vi "KE622x -- Set List Sweep Steps.vi"(0 "Resource In":refnum<visa-resource-name>, 1 "Check For SCPI Errors? (T)":bool=TRUE, 7 "List Sweep Steps In":T1 {"Current Level (A)" min=-0.105 max=0.105 format="%.4p"; "Source Delay (s)" min=0.001 max=1000.0 step=0.001 format="%.3f"; "Voltage Limit (V)" min=0.1 max=105.0 step=0.01 format="%.2p"}, 11 "error in (no error)":errorcluster, 12 "Read Back Set Values? (T)":bool=TRUE) -> (4 "Resource Out (dupl)":refnum<visa-resource-name>, 8 "List Sweep Steps Out":T1 {"Current Level (A)" min=-0.105 max=0.105 format="%.4p"; "Source Delay (s)" min=0.001 max=1000.0 step=0.001 format="%.3f"; "Voltage Limit (V)" min=0.1 max=105.0 step=0.01 format="%.2p"}, 15 "error out":errorcluster)   [LabVIEW 2019, in "Keithley 622x.lvlib"]
doc: "Sets up the individual points in a list current sweep."
uses:
  Keithley 622x.lvlib
  Typedefs/KE622x -- List Sweep Steps.ctl
  Typedefs/KE622x -- List Sweep Step.ctl
  Typedefs/KE622x -- Current Level.ctl
  Typedefs/KE622x -- Source Delay.ctl
  Typedefs/KE622x -- Voltage Limit.ctl
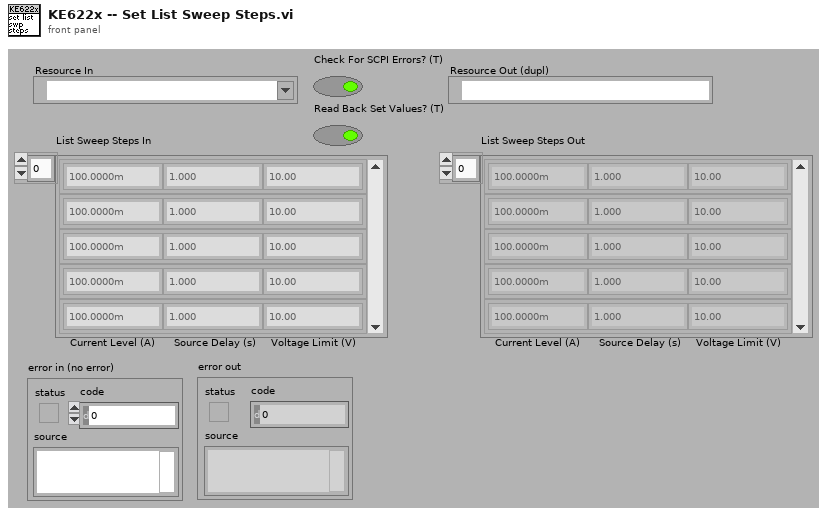
[diagram p1: front panel]
types:
  T1 = typedef "Keithley 622x.lvlib/KE622x -- List Sweep Steps.ctl" = T2[]
  T2 = typedef "Keithley 622x.lvlib/KE622x -- List Sweep Step.ctl" = cluster{"Current Level (A)":T3, "Source Delay (s)":T4, "Voltage Limit (V)":T5}
  T3 = typedef "Keithley 622x.lvlib/KE622x -- Current Level.ctl" = dbl
  T4 = typedef "Keithley 622x.lvlib/KE622x -- Source Delay.ctl" = dbl
  T5 = typedef "Keithley 622x.lvlib/KE622x -- Voltage Limit.ctl" = dbl
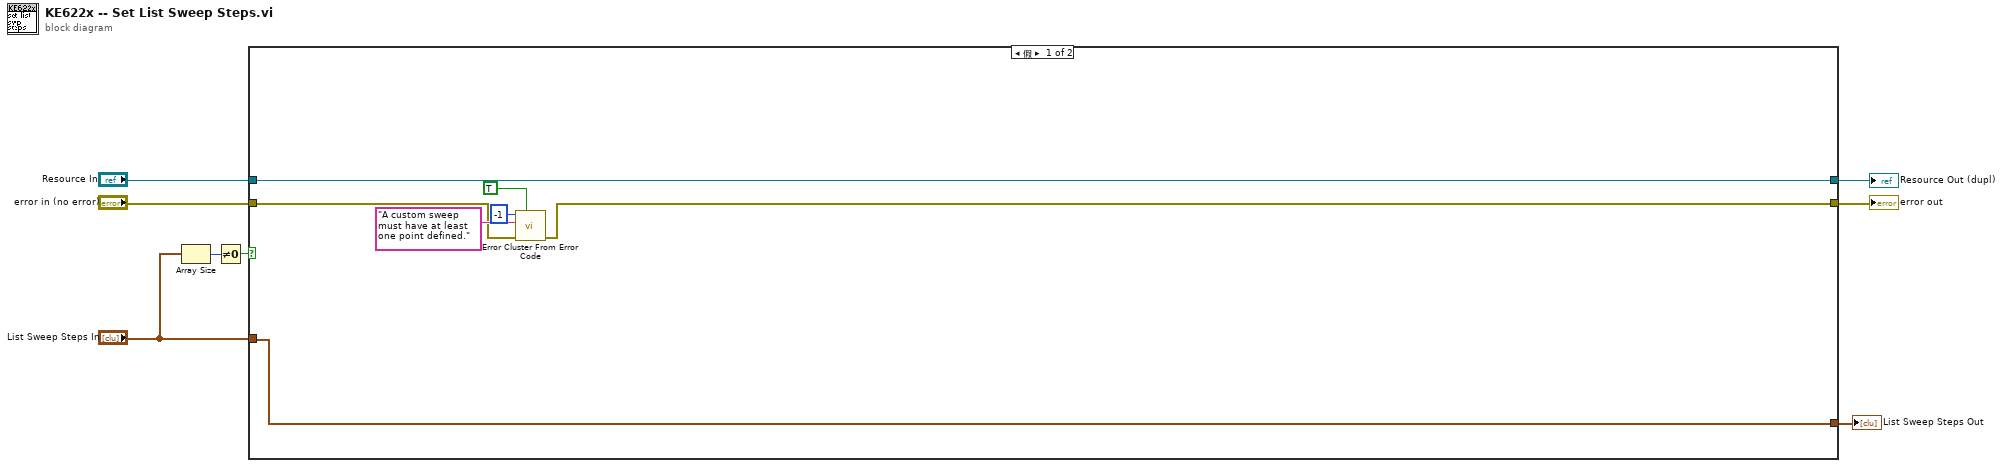
[diagram p0: block diagram]
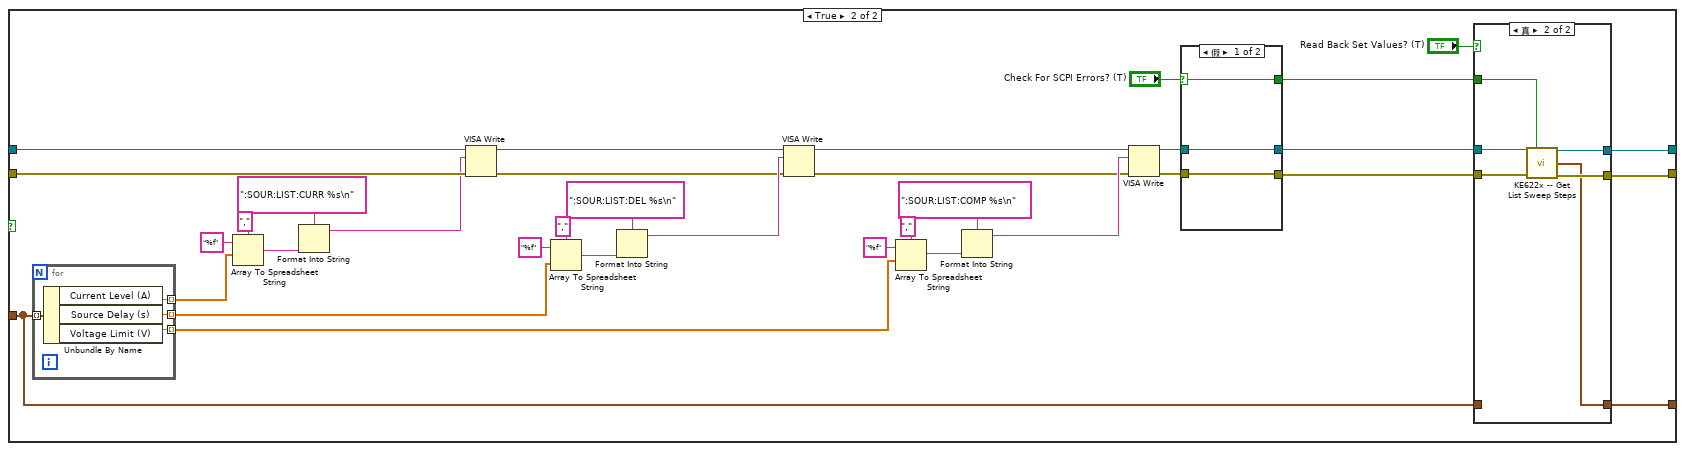
[diagram p2: hidden frame]
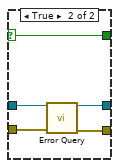
[diagram p4: hidden frame]
diagram:
  n1 = Array Size(array="List Sweep Steps In") -> (size(s)=w6:i32)
  n2 = Not Equal To 0?(x=w6) -> (x != 0?=w5:bool)
  n3 = case shown="假" w5 {
    tunnel: "List Sweep Steps In" -> [w14 w22]
    tunnel: "Resource In" -> [w15 w48]
    tunnel: "error in (no error)" -> [w11 w47]
    tunnel: [w15 w18] -> w3
    tunnel: [w9 w17] -> w2
    tunnel: [w14 w16] -> w1
    frame False {
      n4 = call <vilib>:"Error Cluster From Error Code.vi"("show call chain? (False)"=TRUE, "error in (no error)"=w11, "error message (\"\")"="A custom sweep must have at least one point defined.", "error code (0)"=-1) -> ("error out"=w9:errorcluster)  [unwired: 5 in]
    }
    frame True {
      n5 = for {
        tunnel: w22 -> [w71] mode=indexing
        tunnel: [w70] -> w49 mode=indexing
        tunnel: [w69] -> w38 mode=indexing
        tunnel: [w68] -> w31 mode=indexing
        n6 = Unbundle By Name(w71) -> ("Current Level (A)"=w70:T3, "Source Delay (s)"=w69:T4, "Voltage Limit (V)"=w68:T5)
      }
      n7 = Array To Spreadsheet String(delimiter (Tab)=",", array=w49, 3:"%f" ("format string")) -> (spreadsheet string=w26:string)
      n8 = Format Into String(format string=":SOUR:LIST:CURR %s\n", w26) -> (resulting string=w43:string)  [unwired: 2 in, 1 out]
      n9 = VISA Write(VISA resource name=w48, write buffer=w43, error in (no error)=w47) -> (VISA resource name out=w36:refnum<visa-resource-name>, error out=w37:errorcluster)  [unwired: 1 out]
      n10 = Array To Spreadsheet String(delimiter (Tab)=",", array=w38, 3:"%f" ("format string")) -> (spreadsheet string=w25:string)
      n11 = Format Into String(format string=":SOUR:LIST:DEL %s\n", w25) -> (resulting string=w39:string)  [unwired: 2 in, 1 out]
      n12 = VISA Write(VISA resource name=w36, write buffer=w39, error in (no error)=w37) -> (VISA resource name out=w29:refnum<visa-resource-name>, error out=w30:errorcluster)  [unwired: 1 out]
      n13 = Array To Spreadsheet String(delimiter (Tab)=",", array=w31, 3:"%f" ("format string")) -> (spreadsheet string=w24:string)
      n14 = Format Into String(format string=":SOUR:LIST:COMP %s\n", w24) -> (resulting string=w32:string)  [unwired: 2 in, 1 out]
      n15 = VISA Write(VISA resource name=w29, write buffer=w32, error in (no error)=w30) -> (VISA resource name out=w28:refnum<visa-resource-name>, error out=w27:errorcluster)  [unwired: 1 out]
      n16 = case shown="假" "Check For SCPI Errors? (T)" {
        selector: "Check For SCPI Errors? (T)" -> [w60 w63]
        tunnel: w28 -> [w62 w67]
        tunnel: w27 -> [w61 w66]
        tunnel: [w61 w65] -> w20
        tunnel: [w62 w64] -> w21
        tunnel: [w60 w63] -> w19
        frame False {
        }
        frame True {
          n17 = call "Error Query.vi"("VISA Resource In"=w67, "error in (no error)"=w66) -> ("VISA Resource Out (dupl)"=w64:refnum<visa-resource-name>, "error out"=w65:errorcluster)  [unwired: 10 in, 2 out]
        }
      }
      n18 = case shown="真" "Read Back Set Values? (T)" {
        tunnel: w22 -> [w53 _]
        tunnel: [w53 w54] -> w16
        tunnel: w21 -> [w52 w59]
        tunnel: w20 -> [w51 w58]
        tunnel: w19 -> [_ w57]
        tunnel: [w52 w56] -> w18
        tunnel: [w51 w55] -> w17
        frame False {
        }
        frame True {
          n19 = call "KE622x -- Get List Sweep Steps.vi"("Resource In"=w59, "Check For SCPI Errors? (T)"=w57, "error in (no error)"=w58) -> ("Resource Out (dupl)"=w56:refnum<visa-resource-name>, "List Sweep Steps"=w54:T1, "error out"=w55:errorcluster)  [unwired: 9 in, 1 out]
        }
      }
    }
  }
  "Resource Out (dupl)" <- w3
  "error out" <- w2
  "List Sweep Steps Out" <- w1
